vi "Demo 1 - Image Gallery - Get Image File.vi"(8 "Error In":errorcluster, 11 "Image Path In":path) -> (0 "Error Out":errorcluster, 3 "Image Out":picture)   [LabVIEW 2011]
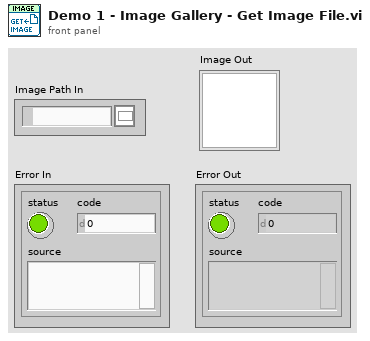
[diagram p1: front panel]
types:
  T1 = typedef "ImageType.ctl" = enum16{"jpg", "png", "bmp"}
  T2 = typedef "imagedata.ctl" = cluster{"image type":i32, "image depth":i32, "image":u8[], "mask":u8[], "colors":u32[], "Rectangle":cluster{"left":i16, "top":i16, "right":i16, "bottom":i16}}
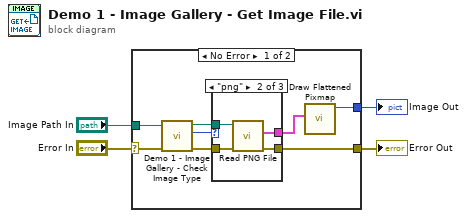
[diagram p0: block diagram]
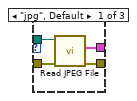
[diagram p2: hidden frame]
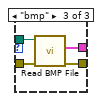
[diagram p3: hidden frame]
diagram:
  n1 = case shown="No Error" "Error In" {
    selector: "Error In" -> [w5 w25]
    tunnel: [w8 _] -> w4
    tunnel: "Image Path In" -> [w7 _]
    tunnel: [w6 w25] -> w2
    frame No Error {
      n2 = call "Demo 1 - Image Gallery - Check Image Type.vi"("error in"=w5, "Image Path In"=w7) -> ("error out"=w12:errorcluster, "Image Type Out"=w11:T1, "Image Path Out"=w10:path)  [unwired: 7 in]
      n3 = case shown="\"png\"" w11 {
        tunnel: w12 -> [w16 w19 w24]
        tunnel: w10 -> [w15 w20 w23]
        tunnel: [w14 w18 w21] -> w9
        tunnel: [w13 w17 w22] -> w6
        frame "jpg", Default {
          n4 = call <vilib>:"Read JPEG File.vi"("error in (no error)"=w16, "path to JPEG file"=w15) -> ("error out"=w13:errorcluster, "image data"=w14:T2)  [unwired: 7 in, 1 out]
        }
        frame "png" {
          n5 = call <vilib>:"Read PNG File.vi"("error in (no error)"=w19, "path to PNG file"=w20) -> ("error out"=w17:errorcluster, "image data"=w18:T2)  [unwired: 7 in, 1 out]
        }
        frame "bmp" {
          n6 = call <vilib>:"Read BMP File.vi"("error in (no error)"=w24, "path to BMP file"=w23) -> ("error out"=w22:errorcluster, "image data"=w21:T2)  [unwired: 7 in, 1 out]
        }
      }
      n7 = call <vilib>:"Draw Flattened Pixmap.vi"("image data"=w9) -> ("new picture"=w8:picture)  [unwired: 8 in]
    }
    frame Error {
    }
  }
  "Image Out" <- w4
  "Error Out" <- w2
